vi "VNA_init.vi"(4 "Stop_Freq(GHz)":dbl=39.5, 5 "HAPS_MCU_CMD":enum16{"Keysight", "R&S"}(ring)=enum."R&S", 6 "Start_Freq(GHz)":dbl=38.5, 7 "sParameter":i32=21, 8 "error in":errorcluster, 9 "SweepPoints":i32=11, 10 "Mark no.":i32=1, 11 "VISA resource name":refnum<visa-resource-name>="TCPIP0::192.168.119.45::inst0::INSTR") -> (0 "error out":errorcluster)   [LabVIEW 2023, in "HAPS.lvlib"]
uses:
  HAPS.lvlib
  Keysight/Keysight.lvlib
  R_S/R_S.lvlib
panel:
  in  "Mark_Freq(GHz)":dbl=39.0
  in  "Step_Freq(GHz)":dbl=0.5 format="%#_13g"
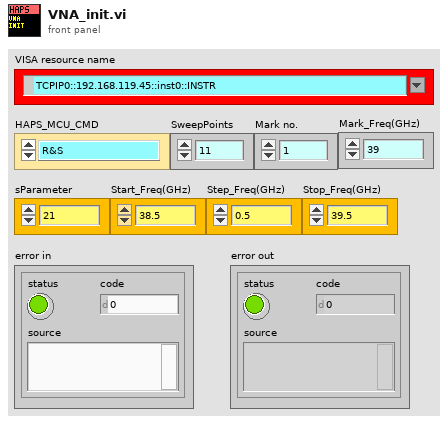
[diagram p1: front panel]
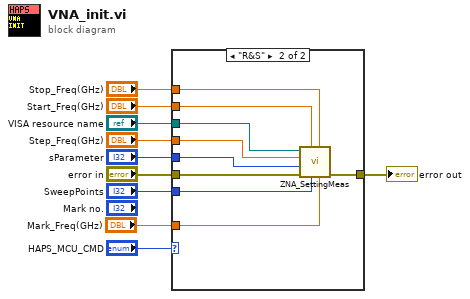
[diagram p0: block diagram]
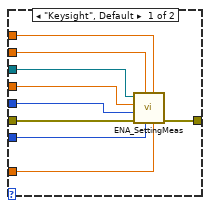
[diagram p2: hidden frame]
diagram:
  n1 = case shown="\"R&S\"" "HAPS_MCU_CMD" {
    tunnel: "sParameter" -> [w19 w26]
    tunnel: "Step_Freq(GHz)" -> [w18 w25]
    tunnel: "VISA resource name" -> [w17 w24]
    tunnel: "Start_Freq(GHz)" -> [w16 w23]
    tunnel: "Stop_Freq(GHz)" -> [w15 w22]
    tunnel: "error in" -> [w14 w28]
    tunnel: [w13 w27] -> w3
    tunnel: "SweepPoints" -> [w12 w21]
    tunnel: "Mark_Freq(GHz)" -> [w11 w20]
    frame "Keysight", Default {
      n2 = call "ENA_SettingMeas.vi"("Mark_Freq(GHz)"=w11, "Stop_Freq(GHz)"=w15, "setSweepPoint"=w12, "Start_Freq(GHz)"=w16, "error in"=w14, "sParameter"=w19, "Step_Freq(GHz)"=w18, "VISA IN"=w17) -> ("error out"=w13:errorcluster)  [unwired: 2 in, 1 out]
    }
    frame "R&S" {
      n3 = call "ZNA_SettingMeas.vi"("Mark_Freq(GHz)"=w20, "Stop_Freq(GHz)"=w22, "SweepPoints"=w21, "Start_Freq(GHz)"=w23, "error in"=w28, "sParameter"=w26, "Step_Freq(GHz)"=w25, "VISA IN"=w24) -> ("error out"=w27:errorcluster)  [unwired: 2 in, 1 out]
    }
  }
  "error out" <- w3
